vi "Main.vi"(8 "error in (no error)":errorcluster) -> ()   [LabVIEW 2017, in "NetworkImpairmentModule.lvlib"]
uses:
  NetworkImpairmentModule.lvlib
  <userlib>/NIST/ModuleAdminLib/ModuleAdmin/ModuleAdmin.lvclass
  C:/Program Files (x86)/National Instruments/LabVIEW 2017/user.lib/NIST/ModuleAdminLib/ModuleAdminBase/ModuleAdminBase.lvclass
  PublicAPI/Arguments/Requests/clStopArgument.ctl
  NetworkImpairmentPlugins/NetworkImpairmentPluginBase_class/NetworkImpairmentPluginBase.lvclass
  C:/Program Files (x86)/National Instruments/LabVIEW 2017/user.lib/NIST/BaseClasses/BasePlugin_class/BasePlugin.lvclass
  <userlib>/NIST/ModuleAdminLib/ModuleAdmin/ModuleAdmin.lvclass/ModuleAdmin.ctl
  <userlib>/NIST/BaseClasses/BasePlugin_class/BasePlugin.lvclass/BasePlugin.ctl
  PublicAPI/Arguments/Requests/dblTimeArray.ctl
  PublicAPI/Arguments/Requests/dblNetImpParams.ctl
  PublicAPI/Arguments/Requests/dblLossThreshold.ctl
  <vilib>/Utility/error.llb/DialogType.ctl
  <userlib>/NIST/ModuleAdminLib/ModuleAdmin/Accessors/Read ShowPanel_.vi
  <userlib>/NIST/ModuleAdminLib/ModuleAdmin/Accessors/Write ShowPanel_.vi
  <userlib>/NIST/BaseClasses/BasePlugin_class/Accessors/Write PluginIniFilePath.vi
  <userlib>/NIST/BaseClasses/BasePlugin_class/Accessors/Read PluginIniFilePath.vi
  <userlib>/NIST/ModuleAdminLib/ModuleAdmin/Accessors/Read CloneRegRef.vi
  <vilib>/Utility/error.llb/Error Cluster From Error Code.vi
  NetworkImpairmentPlugins/NetworkImpairmentPluginBase_class/Accessors/Write TimeArray.vi
  NetworkImpairmentPlugins/NetworkImpairmentPluginBase_class/Accessors/Write NetImpParams.vi
  NetworkImpairmentPlugins/NetworkImpairmentPluginBase_class/Accessors/Read NetImpParams.vi
  NetworkImpairmentPlugins/NetworkImpairmentPluginBase_class/Accessors/Write LossThreshold.vi
  NetworkImpairmentPlugins/NetworkImpairmentPluginBase_class/Accessors/Read LossThreshold.vi
  NetworkImpairmentPlugins/NetworkImpairmentPluginBase_class/Accessors/Get NetworkTime.vi
  NetworkImpairmentPlugins/NetworkImpairmentPluginBase_class/Accessors/Get PktLoss.vi
  <vilib>/ErrorRing/Error Ring.xnode
  <userlib>/NIST/ModuleAdminLib/CloneRegistration/CloneRegistration.lvclass
  <userlib>/NIST/ModuleAdminLib/ModuleAdmin.lvlib
  <userlib>/NIST/BaseClasses/Object_class/BaseObject.lvclass
panel:
  out "error out":errorcluster
  in  "ModuleAdmin":refnum<class "ModuleAdmin.lvclass">
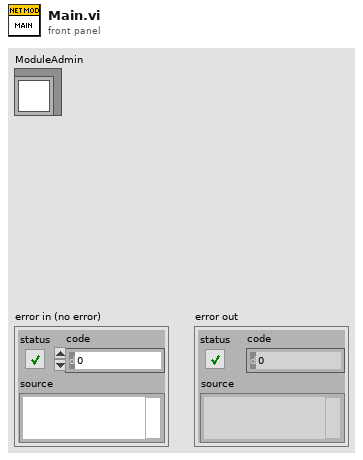
[diagram p1: front panel]
types:
  T1 = typedef "NetworkImpairmentModule.lvlib/clRequestEvents.ctl" = cluster{"StopRequest":refnum<user-event>, "WriteTimeArrayRequest":refnum<user-event>, "WriteNetImpParamsRequest":refnum<user-event>, "ReadNetImpParamsRequest":refnum<user-event>, "WriteLossThresholdRequest":refnum<user-event>, "ReadLossThresholdRequest":refnum<user-event>, "GetNetworkTimeRequest":refnum<user-event>, "GetPktLossRequest":refnum<user-event>, "LoadPluginRequest":refnum<user-event>, "ReadPathToPluginRequest":refnum<user-event>, "ShowPanel":refnum<user-event>}
  T2 = typedef "NetworkImpairmentModule.lvlib/clBroadcastEvents.ctl" = cluster{"DidInit":refnum<user-event>, "StatusUpdate":refnum<user-event>, "ErrorReport":refnum<user-event>, "DidStop":refnum<user-event>, "ReadNetImpParams":refnum<user-event>, "ReadLossThreshold":refnum<user-event>, "GetNetworkTime":refnum<user-event>, "GetPktLoss":refnum<user-event>, "ReadPathToPlugin":refnum<user-event>}
  T3 = typedef "NetworkImpairmentModule.lvlib/clStopArgument.ctl" = cluster{"Exit via Stop Module Req?":bool, "Wait for Module to stop?":bool, "ModuleAdmin":refnum<class "ModuleAdmin.lvclass">}
  T4 = enum32{"Invalid", "Standard", "Closed", "Hidden", "Minimized", "Maximized"}
  T5 = typedef "NetworkImpairmentModule.lvlib/dblTimeArray.ctl" = dbl[]
  T6 = typedef "NetworkImpairmentModule.lvlib/dblNetImpParams.ctl" = dbl[][]
  T7 = typedef "NetworkImpairmentModule.lvlib/dblLossThreshold.ctl" = dbl[]
  T8 = typedef "DialogType.ctl" = u16
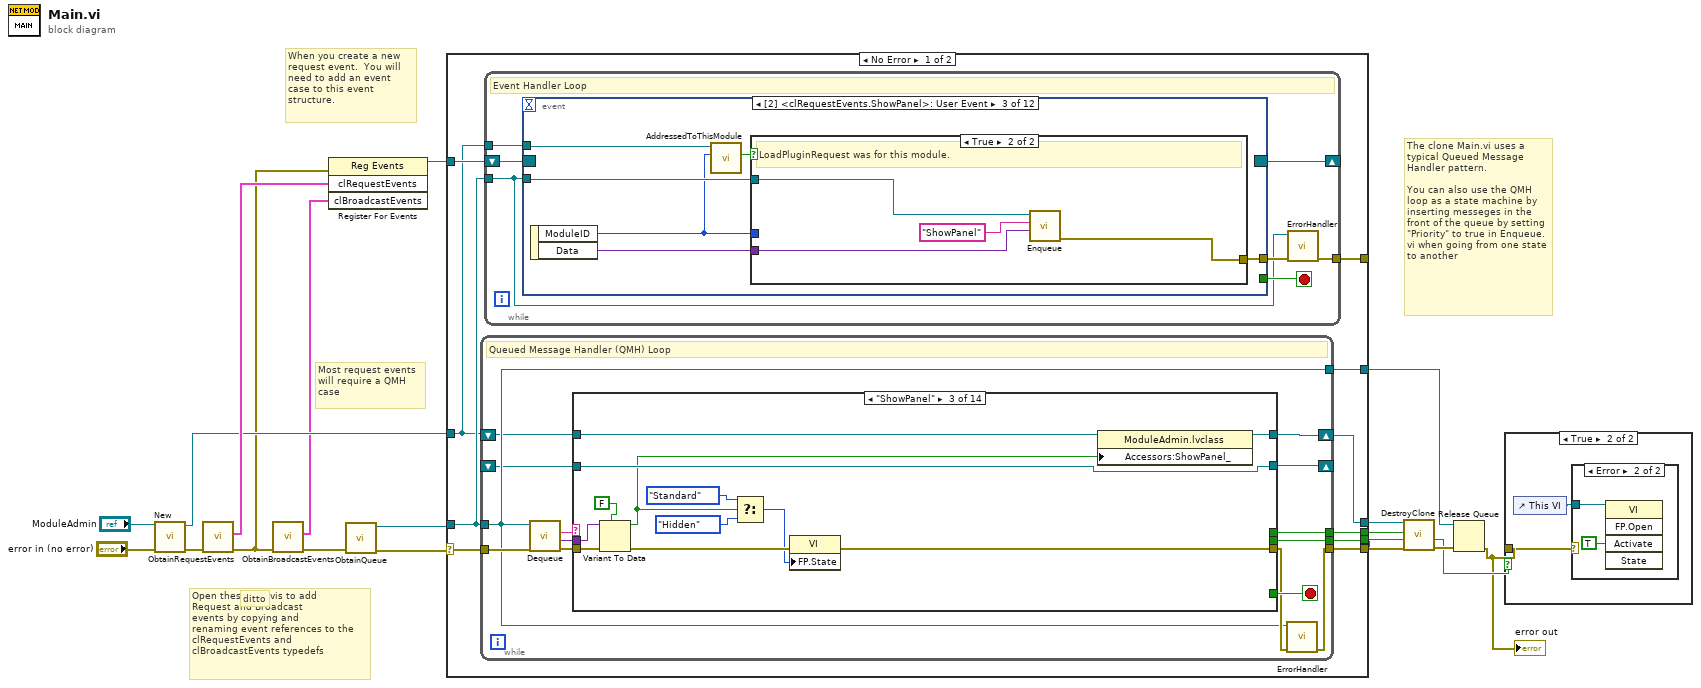
[diagram p0: block diagram]
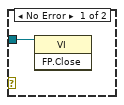
[diagram p3: hidden frame]
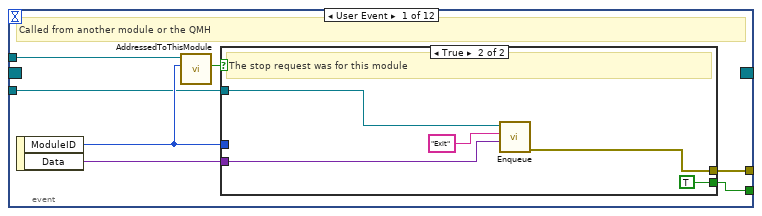
[diagram p4: hidden frame]
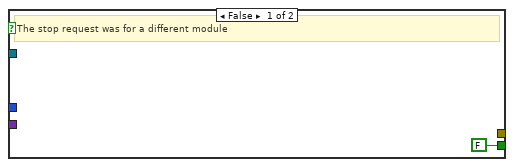
[diagram p5: hidden frame]
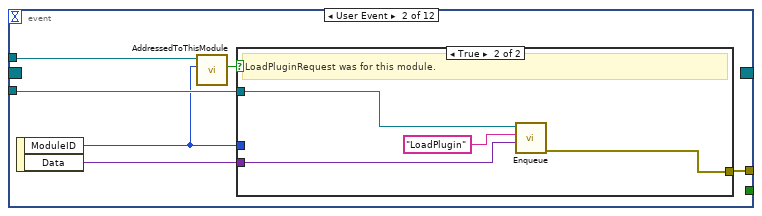
[diagram p6: hidden frame]
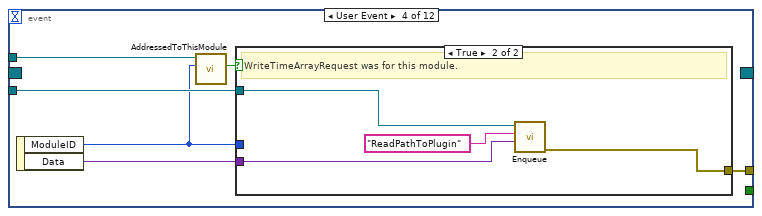
[diagram p9: hidden frame]
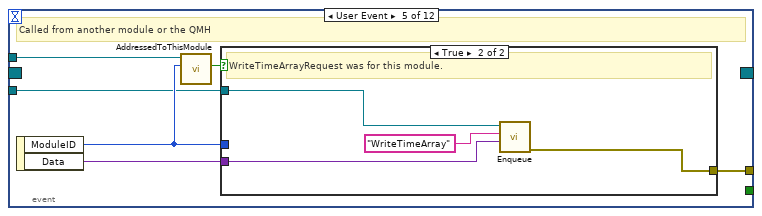
[diagram p11: hidden frame]
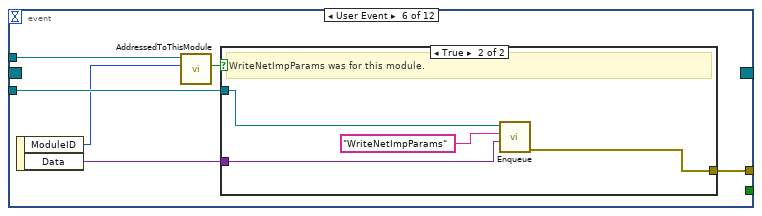
[diagram p13: hidden frame]
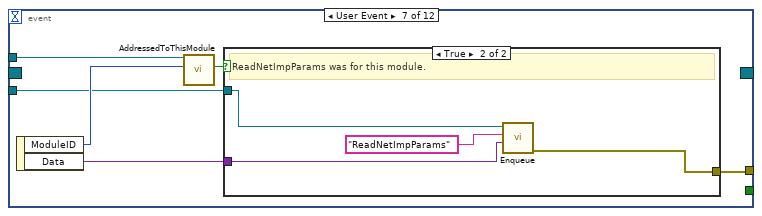
[diagram p15: hidden frame]
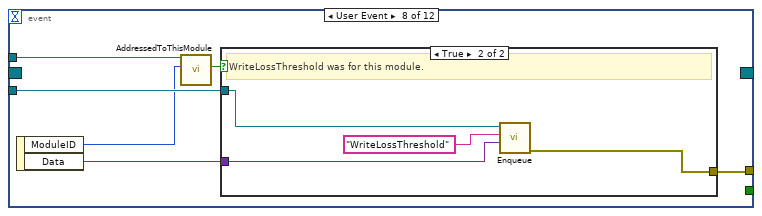
[diagram p17: hidden frame]
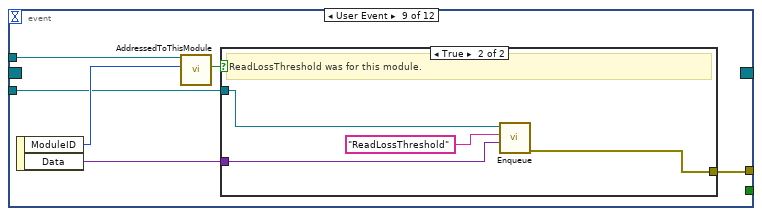
[diagram p19: hidden frame]
diagram:
  # "The clone Main.vi uses a typical Queued Message Handler pattern.  \n\nYou can also use the QMH loop as a state machine by inserting messeges in the front of the queue by setting \"Priority\" to true in Enqueue.vi when going from one state to another"
  # "Open these two vis to add\nRequest and Broadcast \nevents by copying and \nrenaming event references to the \nclRequestEvents and \nclBroadcastEvents typedefs"
  # "ditto"
  # "Most request events\nwill require a QMH\ncase"
  # "When you create a new request event.  You will need to add an event case to this event structure."
  n1 = call <userlib>:"New.vi"("error in (no error)"="error in (no error)", "ModuleAdmin"="ModuleAdmin") -> ("error out"=w17:errorcluster, "ModuleAdmin"=w13:refnum<class "ModuleAdmin.lvclass">)  [unwired: 7 in, 1 out]
  n2 = call "ObtainRequestEvents.vi"("error in (no error)"=w17) -> ("error out"=w10:errorcluster, "clRequestEvents"=w16:T1)  [unwired: 9 in]
  n3 = call "ObtainBroadcastEvents.vi"("error in (no error)"=w10) -> ("error out"=w11:errorcluster, "clBroadcastEvents"=w9:T2)  [unwired: 9 in]
  n4 = register-events(error in=w10, w16, w9) -> (reference out=w8:refnum<event-registration>)  [unwired: 1 in, 1 out]
  n5 = call "ObtainQueue.vi"("error in (no error)"=w11) -> ("error out"=w15:errorcluster, "MessageQueue"=w14:refnum<queue>)  [unwired: 9 in]
  n6 = case shown="No Error" w15 {
    selector: w15 -> [w29 w405]
    tunnel: w14 -> [w27 w401]
    tunnel: w13 -> [w24 w402]
    tunnel: [w28 w403] -> w7
    tunnel: [w26 w401] -> w12
    tunnel: w8 -> [w25 _]
    tunnel: [w23 w400] -> w5
    tunnel: [w22 _] -> w4
    tunnel: [w21 _] -> w3
    tunnel: [w20 _] -> _
    frame No Error {
      n7 = while {
        tunnel: w27 -> [w167]
        tunnel: w29 -> [w175]
        tunnel: [w169] -> w28
        tunnel: [w167] -> w26
        tunnel: [w171] -> w22
        tunnel: [w170] -> w21
        shift-right: [w166] -> _
        shift-left: _ -> [w165]
        shift-right: [w163] -> w23
        shift-left: w24 -> [w164]
        stop <- w176 stop-if-true
        # "Queued Message Handler (QMH) Loop"
        n8 = call "Dequeue.vi"("error in (no error)"=w175, "MessageQueue"=w167) -> ("error out"=w174:errorcluster, "Message Data"=w172:variant, "Message"=w173:string)  [unwired: 6 in, 1 out]
        n9 = case shown="\"ShowPanel\"" w173 {
          selector: w173 -> [w181 _ _ _ _ _ _ _ _ _ _ _ _ _]
          tunnel: [_ _ _ _ _ _ _ _ _ _ _ _ TRUE _] -> w176
          tunnel: w164 -> [w184 w213 w227 w236 w286 w293 w304 w317 w325 w339 w353 w364 w370 w391]
          tunnel: [w180 w202 w228 w242 w283 w291 w302 w319 w323 w337 w347 w360 w377 w382] -> w168
          tunnel: w174 -> [_ _ w233 w244 w284 w299 w306 w316 w326 w341 w350 w362 w376 w390]
          tunnel: w172 -> [_ _ w222 w243 _ w298 w301 _ w327 _ _ _ w375 w389]
          tunnel: [_ _ _ _ _ _ _ _ _ _ _ _ w373 _] -> w171
          tunnel: [_ _ _ _ _ _ _ _ _ _ _ _ w372 _] -> w170
          tunnel: [w178 refnum<class "NetworkImpairmentPluginBase.lvclass"> refnum ("NetworkImpairmentPlugins.lvlib:NetworkImpairmentPluginBase.lvclass") w226 w240 w281 w292 w303 w314 w324 w338 w354 w363 w371 w381] -> w166
          tunnel: w165 -> [w178 _ w226 w245 w285 w296 w305 w321 w329 w340 w352 w365 w371 w381]
          tunnel: [w177 w193 w223 w234 w278 w287 w300 w313 w322 w335 w344 w357 w370 w379] -> w163
          frame Default {
            # "Called only if a message was queued and no QMH case was created"
            n10 = property class="ModuleAdmin.lvclass"(reference=w184) -> (reference out=w177:refnum<class "ModuleAdmin.lvclass">, "Accessors:Module ID"=w183:i32, "Accessors:ModuleName"=w179:string)  [unwired: 1 in, 1 out]
            n11 = call <userlib>:"ModuleName.vi"("Name"=w179, "ModuleID"=w183) -> ("ModuleName"=w182:string)  [unwired: 9 in]
            n12 = xnode "Error Ring"("parameter 0"=w181, "parameter 1"=w182) -> ("error out"=w180:errorcluster)
          }
          frame "Initialize" {
            # "Initialize is always called after ObtainQueue.vi is run"
            n13 = property class="ModuleAdmin.lvclass"(reference=w213) -> (reference out=w198:refnum<class "ModuleAdmin.lvclass">, error out=w210:errorcluster, "Accessors:Module ID"=w201:i32, "Accessors:ShowPanel_"=w196:bool, "Accessors:External Launch"=w195:bool, "Accessors:ModuleName"=w197:string)  [unwired: 1 in]
            n14 = Compound Arithmetic op=OR(w196, invert w195) -> (w194:bool)
            n15 = Select(t=T4."Standard" ("Front Panel Window:State"), s=w194, f=T4."Hidden" ("Front Panel Window:State")) -> (s? t:f=w206:T4)
            n16 = invoke class="VI" method="FP.Open"(error in=w210, "State"=w206) -> (error out=w209:errorcluster)  [unwired: 3 in, 4 out]
            n17 = call <userlib>:"ModuleName.vi"("Name"=w197, "ModuleID"=w201) -> ("ModuleName"=w205:string)  [unwired: 9 in]
            n18 = property class="VI"(error in=w209, "Front Panel.Title"=w205) -> (reference out=w212:refnum<vi>, error out=w211:errorcluster)  [unwired: 1 in]
            n19 = invoke class="VI" method="FP.Center"(reference=w212, error in=w211) -> (error out=w200:errorcluster)  [unwired: 1 in, 2 out]
            n20 = case shown="True" w195 {
              tunnel: [w215 w220] -> w203
              tunnel: [w214 w217] -> w193
              tunnel: w200 -> [w215 w219]
              tunnel: w198 -> [w214 w216]
              frame False {
              }
              frame True {
                n21 = call <userlib>:"WaitOnModuleSync.vi"("error in (no error)"=w219, "ModuleAdmin"=w216) -> ("error out"=w221:errorcluster, "ModuleAdmin"=w218:refnum<class "ModuleAdmin.lvclass">)  [unwired: 8 in]
                n22 = call <userlib>:"WaitOnEventSync.vi"("error in (no error)"=w221, "ModuleAdmin"=w218) -> ("error out"=w220:errorcluster, "ModuleAdmin"=w217:refnum<class "ModuleAdmin.lvclass">)  [unwired: 8 in]
              }
            }
            n23 = call "DidInit.vi"("Init?"=TRUE, "error in (no error)"=w203, "ModuleAdmin"=w193) -> ("error out"=w202:errorcluster)  [unwired: 8 in]
          }
          frame "ShowPanel" {
            n24 = Variant To Data(error in=w233, type=FALSE, Variant=w222) -> (data=w224:bool, error out=w232:errorcluster)
            n25 = Select(t=T4."Standard" ("Front Panel Window:State"), s=w224, f=T4."Hidden" ("Front Panel Window:State")) -> (s? t:f=w225:T4)
            n26 = property class="VI"(error in=w232, "FP.State"=w225) -> (error out=w228:errorcluster)  [unwired: 1 in, 1 out]
            n27 = property class="ModuleAdmin.lvclass"(reference=w227, "Accessors:ShowPanel_"=w224) -> (reference out=w223:refnum<class "ModuleAdmin.lvclass">)  [unwired: 1 in, 1 out]
          }
          frame "LoadPlugin" {
            # "Load the plugin and store the INI file path in NetworkPluginBase class."
            n28 = Variant To Data(error in=w244, type=path "", Variant=w243) -> (data=w235:path, error out=w250:errorcluster)
            n29 = call <userlib>:"GetPathToClass.vi"("error in (no error)"=w250, "configuration file path"=w235) -> ("error IO"=w249:errorcluster, "PathToClass"=w238:path)  [unwired: 8 in]
            n30 = Current VI's Path() -> (path=w239:path)
            n31 = Build Path(base path=w239, name or relative path=w238) -> (appended path=w237:path)
            n32 = call <vilib>:"Check if File or Folder Exists.vi"("error in (no error)"=w249, "path"=w237) -> ("error out"=w247:errorcluster, "file or folder exists?"=w248:bool, "dup path"=w246:path)  [unwired: 7 in]
            n33 = case shown="False" w248 {
              tunnel: w246 -> [w255 w265]
              tunnel: w247 -> [w263 w270]
              tunnel: [w259 w268] -> w242
              tunnel: w245 -> [_ w269]
              tunnel: [w256 w269] -> w241
              tunnel: w236 -> [w254 w264]
              tunnel: [w252 w264] -> w234
              frame True {
                n34 = property class="ModuleAdmin.lvclass"(reference=w254) -> (reference out=w252:refnum<class "ModuleAdmin.lvclass">, "Accessors:Module ID"=w253:i32)  [unwired: 1 in, 1 out]
                n35 = call-dynamic "LoadClassFromFile.vi"("error in (no error)"=w263, "class path"=w255, "reference in"=refnum<class "NetworkImpairmentPluginBase.lvclass"> refnum ("NetworkImpairmentPlugins.lvlib:NetworkImpairmentPluginBase.lvclass")) -> ("error out"=w258:errorcluster, "reference out"=w256:refnum<class "NetworkImpairmentPluginBase.lvclass">)  [unwired: 7 in]
                n36 = Path To String(path=w255) -> (string=w261:string)
                n37 = Format Into String(format string="Plugin %s loaded", w261) -> (resulting string=w257:string)  [unwired: 2 in, 1 out]
                n38 = call "StatusUpdate.vi"("error in (no error)"=w258, "Status"=w257, "ModuleID"=w253) -> ("error out"=w259:errorcluster)  [unwired: 8 in]
              }
              frame False {
                n39 = Path To String(path=w265) -> (string=w266:string)
                n40 = xnode "Error Ring"("parameter 0"=w266) -> ("error out"=w267:errorcluster)
                n41 = Merge Errors(w267, w270) -> (w268:errorcluster)
              }
            }
            n42 = property class="NetworkImpairmentPluginBase.lvc"(reference=w241, "Accessors:PluginIniFilePath"=w235) -> (reference out=w240:refnum<class "NetworkImpairmentPluginBase.lvclass">)  [unwired: 1 in, 1 out]
          }
          frame "ReadPathToPlugin" {
            # "Read INI file path from NetworkPluginBase class."
            n43 = property class="NetworkImpairmentPluginBase.lvc"(reference=w285, error in=w284) -> (reference out=w281:refnum<class "NetworkImpairmentPluginBase.lvclass">, error out=w280:errorcluster, "Accessors:PluginIniFilePath"=w279:path)
            n44 = property class="ModuleAdmin.lvclass"(reference=w286) -> (reference out=w278:refnum<class "ModuleAdmin.lvclass">, "Accessors:Module ID"=w282:i32)  [unwired: 1 in, 1 out]
            n45 = call "ReadPathToPlugin.vi"("error in (no error)"=w280, "Path"=w279, "ModuleID"=w282) -> ("error out"=w283:errorcluster)  [unwired: 8 in]
          }
          frame "WriteTimeArray" {
            w297 = T5 []  # TimeArray
            # "Write the Time Array from the Event Module to the Network Impairment Module for impairment."
            n46 = Variant To Data(error in=w299, type=w297, Variant=w298) -> (data=w294:T5, error out=w295:errorcluster)
            n47 = property class="NetworkImpairmentPluginBase.lvc"(reference=w296, error in=w295, "Accessors:dblTimeArray"=w294) -> (reference out=w292:refnum<class "NetworkImpairmentPluginBase.lvclass">, error out=w289:errorcluster)
            n48 = property class="ModuleAdmin.lvclass"(reference=w293) -> (reference out=w287:refnum<class "ModuleAdmin.lvclass">, "Accessors:Module ID"=w290:i32)  [unwired: 1 in, 1 out]
            n49 = call "StatusUpdate.vi"("error in (no error)"=w289, "Status"="Time Array Received", "ModuleID"=w290) -> ("error out"=w291:errorcluster)  [unwired: 8 in]
          }
          frame "WriteNetImpParams" {
            w312 = T6 []  # dblNetImpParams
            # "Write Network Impairment Parameters to the module."
            n50 = Variant To Data(error in=w306, type=w312, Variant=w301) -> (data=w310:T6, error out=w311:errorcluster)
            n51 = property class="NetworkImpairmentPluginBase.lvc"(reference=w305, error in=w311, "Accessors:dblNetImpParams"=w310) -> (reference out=w303:refnum<class "NetworkImpairmentPluginBase.lvclass">, error out=w308:errorcluster)
            n52 = property class="ModuleAdmin.lvclass"(reference=w304) -> (reference out=w300:refnum<class "ModuleAdmin.lvclass">, "Accessors:Module ID"=w309:i32)  [unwired: 1 in, 1 out]
            n53 = call "StatusUpdate.vi"("error in (no error)"=w308, "Status"="Impairment Parameters Received", "ModuleID"=w309) -> ("error out"=w302:errorcluster)  [unwired: 8 in]
          }
          frame "ReadNetImpParams" {
            # "Broadcast the Network Impairment Parameters as a user event."
            n54 = property class="NetworkImpairmentPluginBase.lvc"(reference=w321, error in=w316) -> (reference out=w314:refnum<class "NetworkImpairmentPluginBase.lvclass">, error out=w315:errorcluster, "Accessors:dblNetImpParams"=w320:dbl[][])
            n55 = property class="ModuleAdmin.lvclass"(reference=w317) -> (reference out=w313:refnum<class "ModuleAdmin.lvclass">, "Accessors:Module ID"=w318:i32)  [unwired: 1 in, 1 out]
            n56 = call "ReadNetImpParams.vi"("error in (no error)"=w315, "dblNetImpParams"=w320, "ModuleID"=w318) -> ("error out"=w319:errorcluster)  [unwired: 8 in]
          }
          frame "WriteLossThreshold" {
            w334 = T7 []  # dblLossThreshold
            # "Write Loss Threshold to Network Impairment module."
            n57 = Variant To Data(error in=w326, type=w334, Variant=w327) -> (data=w328:T7, error out=w333:errorcluster)
            n58 = property class="NetworkImpairmentPluginBase.lvc"(reference=w329, error in=w333, "Accessors:dblLossThreshold"=w328) -> (reference out=w324:refnum<class "NetworkImpairmentPluginBase.lvclass">, error out=w331:errorcluster)
            n59 = property class="ModuleAdmin.lvclass"(reference=w325) -> (reference out=w322:refnum<class "ModuleAdmin.lvclass">, "Accessors:Module ID"=w332:i32)  [unwired: 1 in, 1 out]
            n60 = call "StatusUpdate.vi"("error in (no error)"=w331, "Status"=" Loss Threshold Received", "ModuleID"=w332) -> ("error out"=w323:errorcluster)  [unwired: 8 in]
          }
          frame "ReadLossThreshold" {
            # "Read Loss Threshold from Network Impairment module."
            n61 = property class="NetworkImpairmentPluginBase.lvc"(reference=w340, error in=w341) -> (reference out=w338:refnum<class "NetworkImpairmentPluginBase.lvclass">, error out=w342:errorcluster, "Accessors:dblLossThreshold"=w336:dbl[])
            n62 = property class="ModuleAdmin.lvclass"(reference=w339) -> (reference out=w335:refnum<class "ModuleAdmin.lvclass">, "Accessors:Module ID"=w343:i32)  [unwired: 1 in, 1 out]
            n63 = call "ReadLossThreshold.vi"("error in (no error)"=w342, "dblLossThreshold"=w336, "ModuleID"=w343) -> ("error out"=w337:errorcluster)  [unwired: 8 in]
          }
          frame "GetNetTime" {
            # "Get Network Time which is impaired using the Network Impairment Plugin \"GetNetTime.vi\"."
            n64 = call-dynamic "GetNetworkTime.vi"("error in (no error)"=w350, "NetworkImpairmentPluginBase in"=w352) -> ("error out"=w349:errorcluster, "NetworkImpairmentPluginBase out"=w351:refnum<class "NetworkImpairmentPluginBase.lvclass">)  [unwired: 8 in]
            n65 = property class="NetworkImpairmentPluginBase.lvc"(reference=w351, error in=w349) -> (reference out=w354:refnum<class "NetworkImpairmentPluginBase.lvclass">, error out=w355:errorcluster, "Accessors:dblNetworkTime"=w356:dbl[])
            n66 = property class="ModuleAdmin.lvclass"(reference=w353) -> (reference out=w344:refnum<class "ModuleAdmin.lvclass">, "Accessors:Module ID"=w346:i32)  [unwired: 1 in, 1 out]
            n67 = call "GetNetTime.vi"("error in (no error)"=w355, "dblNetTime"=w356, "ModuleID"=w346) -> ("error out"=w348:errorcluster)  [unwired: 8 in]
            n68 = call "StatusUpdate.vi"("error in (no error)"=w348, "Status"="Net Impairment Time Transmitted", "ModuleID"=w346) -> ("error out"=w347:errorcluster)  [unwired: 8 in]
          }
          frame "GetPktLoss" {
            # "Get Packet Loss data which is generated using Network Impairment Plugin \"GetPktLoss.vi\"."
            n69 = call-dynamic "GetPktLoss.vi"("error in (no error)"=w362, "NetworkImpairmentPluginBase in"=w365) -> ("error out"=w366:errorcluster, "NetworkImpairmentPluginBase out"=w367:refnum<class "NetworkImpairmentPluginBase.lvclass">)  [unwired: 8 in]
            n70 = property class="NetworkImpairmentPluginBase.lvc"(reference=w367, error in=w366) -> (reference out=w363:refnum<class "NetworkImpairmentPluginBase.lvclass">, error out=w368:errorcluster, "Accessors:dblPktLoss"=w369:dbl[])
            n71 = property class="ModuleAdmin.lvclass"(reference=w364) -> (reference out=w357:refnum<class "ModuleAdmin.lvclass">, "Accessors:Module ID"=w359:i32)  [unwired: 1 in, 1 out]
            n72 = call "GetPktLoss.vi"("error in (no error)"=w368, "dblPktLoss"=w369, "ModuleID"=w359) -> ("error out"=w361:errorcluster)  [unwired: 8 in]
            n73 = call "StatusUpdate.vi"("error in (no error)"=w361, "Status"="Net Pkt Loss Transmitted", "ModuleID"=w359) -> ("error out"=w360:errorcluster)  [unwired: 8 in]
          }
          frame "Exit" {
            # "Called by the StopRequest event handler case"
            n74 = control-ref of="This VI"() -> (w374:refnum<vi>)
            n75 = call "HandleExit.vi"("error in (no error)"=w376, "VI Refnum"=w374, "StopArgument"=w375, "ModuleAdmin"=w370) -> ("error out"=w377:errorcluster, "Exit via Stop Module Req?"=w372:bool, "WaitForStop?"=w373:bool)  [unwired: 5 in]
          }
          frame "Error" {
            n76 = property class="ModuleAdmin.lvclass"(reference=w391) -> (reference out=w380:refnum<class "ModuleAdmin.lvclass">, "Accessors:External Launch"=w385:bool, "Accessors:Module ID"=w383:i32)  [unwired: 1 in, 1 out]
            n77 = Variant To Data(error in=w390, type=errorcluster {"status"=FALSE, "code"=0, "source"=""} ("error constant"), Variant=w389) -> (data=w384:errorcluster, error out=w387:errorcluster)
            n78 = call "ReportError.vi"("error in (no error)"=w387, "ErrorReported"=w384, "ModuleID"=w383) -> ("error out"=w386:errorcluster)  [unwired: 8 in]
            n79 = case shown="False" w385 {
              tunnel: w386 -> [w395 w397]
              tunnel: w384 -> [w394 _]
              tunnel: [w393 w397] -> w382
              tunnel: w380 -> [w392 w396]
              tunnel: [w392 w396] -> w379
              frame False {
                # "Todo:  Add an event to ask the user\nIf the module should stop or continue"
                # "Stand alone: now, force an exit"
                n80 = call <vilib>:"Simple Error Handler.vi"("error in (no error)"=w394) -> ()  [unwired: 4 in, 5 out]
                n81 = call "StopRequest.vi"("error in (no error)"=w395, "ModuleAdmin"=w392) -> ("error out"=w393:errorcluster)  [unwired: 8 in, 1 out]
              }
              frame True {
                # "Externally launched modules only broadcast the error msg"
              }
            }
          }
        }
        n82 = call "ErrorHandler.vi"("error in (no error)"=w168, "MessageQueue"=w167) -> ("error out"=w169:errorcluster)  [unwired: 8 in, 1 out]
      }
      n83 = while {
        tunnel: w27 -> [w30]
        shift-right: [w34] -> _
        shift-left: w25 -> [w35]
        tunnel: w24 -> [w33]
        tunnel: [w31] -> w20
        stop <- w36 stop-if-true
        # "Event Handler Loop"
        n84 = event shown="[2] <clRequestEvents.ShowPanel>: User Event" {
          selector: w35 -> [_ _ _ _ _ _ _ _ _ _ _ _]
          dyn-events: [_ _ _ _ _ _ _ _ _ _ _ _] -> w34
          timeout: _ -> [_ _ _ _ _ _ _ _ _ _ _ _]
          tunnel: w30 -> [w40 w54 w64 w73 w82 w93 w101 w113 w122 w131 w142 w162]
          tunnel: [w39 _ _ _ _ _ _ _ _ _ _ TRUE] -> w36
          tunnel: w33 -> [w43 w53 w63 w74 w85 w94 w102 w114 w123 w132 w144 w156]
          tunnel: [w38 w50 w60 w70 w81 w90 w100 w110 w120 w130 w140 w160] -> w32
          event User Event {
            # "Called from another module or the QMH"
            n85 = event-data() -> ("ModuleID"=w41:i32, "Data"=w37:variant)  [unwired: 1 in]
            n86 = call <userlib>:"AddressedToThisModule.vi"("ModuleID"=w41, "ModuleAdmin"=w43) -> ("AddressedToThisInstance?"=w42:bool)  [unwired: 8 in, 1 out]
            n87 = case shown="True" w42 {
              tunnel: w41 -> [_ _]
              tunnel: w40 -> [_ w49]
              tunnel: [FALSE TRUE] -> w39
              tunnel: [_ w47] -> w38
              tunnel: w37 -> [_ w45]
              frame False {
                # "The stop request was for a different module"
              }
              frame True {
                # "The stop request was for this module"
                n88 = call "Enqueue.vi"("Message Data"=w45, "Message"="Exit", "MessageQueue"=w49) -> ("error out"=w47:errorcluster)  [unwired: 7 in, 1 out]
              }
            }
          }
          event User Event {
            n89 = event-data() -> ("ModuleID"=w52:i32, "Data"=w51:variant)  [unwired: 1 in]
            n90 = call <userlib>:"AddressedToThisModule.vi"("ModuleID"=w52, "ModuleAdmin"=w53) -> ("AddressedToThisInstance?"=w55:bool)  [unwired: 8 in, 1 out]
            n91 = case shown="True" w55 {
              tunnel: w52 -> [_ _]
              tunnel: w54 -> [_ w59]
              tunnel: [_ w58] -> w50
              tunnel: w51 -> [_ w56]
              frame False {
                # "The request was not for this module."
              }
              frame True {
                # "LoadPluginRequest was for this module."
                n92 = call "Enqueue.vi"("Message Data"=w56, "Message"="LoadPlugin", "MessageQueue"=w59) -> ("error out"=w58:errorcluster)  [unwired: 7 in, 1 out]
              }
            }
          }
          event User Event {
            n93 = event-data() -> ("ModuleID"=w62:i32, "Data"=w61:variant)  [unwired: 1 in]
            n94 = call <userlib>:"AddressedToThisModule.vi"("ModuleID"=w62, "ModuleAdmin"=w63) -> ("AddressedToThisInstance?"=w65:bool)  [unwired: 8 in, 1 out]
            n95 = case shown="True" w65 {
              tunnel: w62 -> [_ _]
              tunnel: w64 -> [_ w69]
              tunnel: [_ w68] -> w60
              tunnel: w61 -> [_ w66]
              frame False {
                # "The request was not for this module."
              }
              frame True {
                # "LoadPluginRequest was for this module."
                n96 = call "Enqueue.vi"("Message Data"=w66, "Message"="ShowPanel", "MessageQueue"=w69) -> ("error out"=w68:errorcluster)  [unwired: 7 in, 1 out]
              }
            }
          }
          event User Event {
            n97 = event-data() -> ("ModuleID"=w72:i32, "Data"=w71:variant)  [unwired: 1 in]
            n98 = call <userlib>:"AddressedToThisModule.vi"("ModuleID"=w72, "ModuleAdmin"=w74) -> ("AddressedToThisInstance?"=w75:bool)  [unwired: 8 in, 1 out]
            n99 = case shown="True" w75 {
              tunnel: w72 -> [_ _]
              tunnel: w73 -> [_ w79]
              tunnel: [_ w78] -> w70
              tunnel: w71 -> [_ w76]
              frame False {
                # "The request was not for this module."
              }
              frame True {
                # "WriteTimeArrayRequest was for this module."
                n100 = call "Enqueue.vi"("Message Data"=w76, "Message"="ReadPathToPlugin", "MessageQueue"=w79) -> ("error out"=w78:errorcluster)  [unwired: 7 in, 1 out]
              }
            }
          }
          event User Event {
            # "Called from another module or the QMH"
            n101 = event-data() -> ("ModuleID"=w83:i32, "Data"=w80:variant)  [unwired: 1 in]
            n102 = call <userlib>:"AddressedToThisModule.vi"("ModuleID"=w83, "ModuleAdmin"=w85) -> ("AddressedToThisInstance?"=w84:bool)  [unwired: 8 in, 1 out]
            n103 = case shown="True" w84 {
              tunnel: w83 -> [_ _]
              tunnel: w82 -> [_ w89]
              tunnel: [_ w88] -> w81
              tunnel: w80 -> [_ w86]
              frame False {
                # "The request was not for this module."
              }
              frame True {
                # "WriteTimeArrayRequest was for this module."
                n104 = call "Enqueue.vi"("Message Data"=w86, "Message"="WriteTimeArray", "MessageQueue"=w89) -> ("error out"=w88:errorcluster)  [unwired: 7 in, 1 out]
              }
            }
          }
          event User Event {
            n105 = event-data() -> ("ModuleID"=w92:i32, "Data"=w91:variant)  [unwired: 1 in]
            n106 = call <userlib>:"AddressedToThisModule.vi"("ModuleID"=w92, "ModuleAdmin"=w94) -> ("AddressedToThisInstance?"=w95:bool)  [unwired: 8 in, 1 out]
            n107 = case shown="True" w95 {
              tunnel: [_ w99] -> w90
              tunnel: w93 -> [_ w97]
              tunnel: w91 -> [_ w96]
              frame False {
                # "The request was not for this module."
              }
              frame True {
                # "WriteNetImpParams was for this module."
                n108 = call "Enqueue.vi"("Message Data"=w96, "Message"="WriteNetImpParams", "MessageQueue"=w97) -> ("error out"=w99:errorcluster)  [unwired: 7 in, 1 out]
              }
            }
          }
          event User Event {
            n109 = event-data() -> ("ModuleID"=w103:i32, "Data"=w104:variant)  [unwired: 1 in]
            n110 = call <userlib>:"AddressedToThisModule.vi"("ModuleID"=w103, "ModuleAdmin"=w102) -> ("AddressedToThisInstance?"=w105:bool)  [unwired: 8 in, 1 out]
            n111 = case shown="True" w105 {
              tunnel: [_ w109] -> w100
              tunnel: w104 -> [_ w107]
              tunnel: w101 -> [_ w106]
              frame False {
                # "The request was not for this module."
              }
              frame True {
                # "ReadNetImpParams was for this module."
                n112 = call "Enqueue.vi"("Message Data"=w107, "Message"="ReadNetImpParams", "MessageQueue"=w106) -> ("error out"=w109:errorcluster)  [unwired: 7 in, 1 out]
              }
            }
          }
          event User Event {
            n113 = event-data() -> ("ModuleID"=w112:i32, "Data"=w111:variant)  [unwired: 1 in]
            n114 = call <userlib>:"AddressedToThisModule.vi"("ModuleID"=w112, "ModuleAdmin"=w114) -> ("AddressedToThisInstance?"=w115:bool)  [unwired: 8 in, 1 out]
            n115 = case shown="True" w115 {
              tunnel: [_ w119] -> w110
              tunnel: w113 -> [_ w117]
              tunnel: w111 -> [_ w116]
              frame False {
                # "The request was not for this module."
              }
              frame True {
                # "WriteLossThreshold was for this module."
                n116 = call "Enqueue.vi"("Message Data"=w116, "Message"="WriteLossThreshold", "MessageQueue"=w117) -> ("error out"=w119:errorcluster)  [unwired: 7 in, 1 out]
              }
            }
          }
          event User Event {
            n117 = event-data() -> ("ModuleID"=w124:i32, "Data"=w121:variant)  [unwired: 1 in]
            n118 = call <userlib>:"AddressedToThisModule.vi"("ModuleID"=w124, "ModuleAdmin"=w123) -> ("AddressedToThisInstance?"=w125:bool)  [unwired: 8 in, 1 out]
            n119 = case shown="True" w125 {
              tunnel: [_ w129] -> w120
              tunnel: w122 -> [_ w127]
              tunnel: w121 -> [_ w126]
              frame False {
                # "The request was not for this module."
              }
              frame True {
                # "ReadLossThreshold was for this module."
                n120 = call "Enqueue.vi"("Message Data"=w126, "Message"="ReadLossThreshold", "MessageQueue"=w127) -> ("error out"=w129:errorcluster)  [unwired: 7 in, 1 out]
              }
            }
          }
          event User Event {
            n121 = event-data() -> ("ModuleID"=w134:i32, "Data"=w133:variant)  [unwired: 1 in]
            n122 = call <userlib>:"AddressedToThisModule.vi"("ModuleID"=w134, "ModuleAdmin"=w132) -> ("AddressedToThisInstance?"=w135:bool)  [unwired: 8 in, 1 out]
            n123 = case shown="True" w135 {
              tunnel: [_ w139] -> w130
              tunnel: w133 -> [_ w137]
              tunnel: w131 -> [_ w136]
              frame False {
                # "The request was not for this module."
              }
              frame True {
                # "GetNetTime was for this module."
                n124 = call "Enqueue.vi"("Message Data"=w137, "Message"="GetNetTime", "MessageQueue"=w136) -> ("error out"=w139:errorcluster)  [unwired: 7 in, 1 out]
              }
            }
          }
          event User Event {
            n125 = event-data() -> ("ModuleID"=w143:i32, "Data"=w141:variant)  [unwired: 1 in]
            n126 = call <userlib>:"AddressedToThisModule.vi"("ModuleID"=w143, "ModuleAdmin"=w144) -> ("AddressedToThisInstance?"=w145:bool)  [unwired: 8 in, 1 out]
            n127 = case shown="True" w145 {
              tunnel: [_ w149] -> w140
              tunnel: w142 -> [_ w147]
              tunnel: w141 -> [_ w146]
              frame False {
                # "The request was not for this module."
              }
              frame True {
                # "GetPktLoss was for this module."
                n128 = call "Enqueue.vi"("Message Data"=w146, "Message"="GetPktLoss", "MessageQueue"=w147) -> ("error out"=w149:errorcluster)  [unwired: 7 in, 1 out]
              }
            }
          }
          event Panel Close? {
            # "Hide on external launch"
            # "Discard the event so the QMH can complete"
            # "Called from another module or the QMH"
            n129 = event-data() -> ()  [unwired: 1 in, 1 out]
            n130 = property class="ModuleAdmin.lvclass"(reference=w156) -> ("Accessors:External Launch"=w151:bool)  [unwired: 1 in, 2 out]
            n131 = Bundle By Name(cluster=T3 {"Exit via Stop Module Req?"=FALSE, "Wait for Module to stop?"=FALSE, "ModuleAdmin"=refnum} ("Stop Argument"), "Wait for Module to stop?"=FALSE, "Exit via Stop Module Req?"=TRUE) -> (w157:T3)
            n132 = Select(t="HidePanel", s=w151, f="Exit" ("Message")) -> (s? t:f=w153:string)
            n133 = call "Enqueue.vi"("Message Data"=w157, "Message"=w153, "MessageQueue"=w162) -> ("error out"=w160:errorcluster)  [unwired: 7 in, 1 out]
            n134 = event-data("Discard?"=TRUE) -> ()  [unwired: 1 in, 1 out]
          }
        }
        n135 = call "ErrorHandler.vi"("error in (no error)"=w32, "MessageQueue"=w30) -> ("error out"=w31:errorcluster)  [unwired: 8 in, 1 out]
      }
    }
    frame Error {
      n136 = property class="ModuleAdmin.lvclass"(reference=w402) -> (reference out=w400:refnum<class "ModuleAdmin.lvclass">, "Accessors:CloneRegRef"=w399:refnum<data-value>, "Accessors:Module ID"=w398:i32)  [unwired: 1 in, 1 out]
      n137 = call <userlib>:"Remove.vi"("Module ID"=w398, "CloneRegRef"=w399) -> ("error out"=w404:errorcluster)  [unwired: 7 in, 2 out]
      n138 = flat-sequence {
        tunnel: w405 -> [w408]
        tunnel: w404 -> [_]
        tunnel: [w406] -> w403
        frame #0 {
          w407 = T8 2 items=["no dialog", "OK message", "continue or stop message", "OK message + warnings", "continue/stop + warnings"] ("type of dialog (OK msg:1)")
          n139 = call <vilib>:"Simple Error Handler.vi"("type of dialog (OK msg:1)"=w407, "error in (no error)"=w408) -> ("error out"=w406:errorcluster)  [unwired: 3 in, 4 out]
        }
      }
    }
  }
  n140 = call "DestroyClone.vi"("error in (no error)"=w7, "Exit via Stop Module Req?"=w3, "Wait for Module to stop?"=w4, "ModuleAdmin"=w5) -> ("error out"=w6:errorcluster, "External Launch"=w2:bool)  [unwired: 5 in, 1 out]
  n141 = Release Queue(queue=w12, error in (no error)=w6) -> (error out=w1:errorcluster)  [unwired: 1 in, 2 out]
  "error out" <- w1
  n142 = case shown="True" w2 {
    tunnel: w1 -> [_ w410]
    frame False {
    }
    frame True {
      n143 = control-ref of="This VI"() -> (w409:refnum<vi>)
      n144 = case shown="Error" w410 {
        tunnel: w409 -> [w411 w412]
        frame No Error {
          n145 = invoke class="VI" method="FP.Close"(reference=w411) -> ()  [unwired: 2 in, 3 out]
        }
        frame Error {
          n146 = invoke class="VI" method="FP.Open"(reference=w412, "Activate"=TRUE ("Activate?")) -> ()  [unwired: 3 in, 5 out]
        }
      }
    }
  }
